vi "Set Variant.vi"(8 "error in (no error)":errorcluster, 10 "Variant":variant, 11 "int32 in":refnum<class "float.lvclass">) -> (0 "error out":errorcluster, 3 "int32 out":refnum<class "float.lvclass">)   [LabVIEW 2020, in "Protobuf RAW.lvlib" / "float.lvclass"]
uses:
  float.lvclass
  float.lvclass/float.ctl
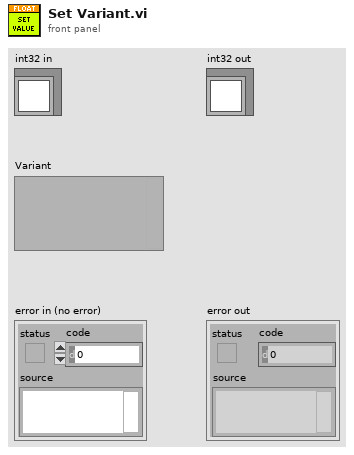
[diagram p1: front panel]
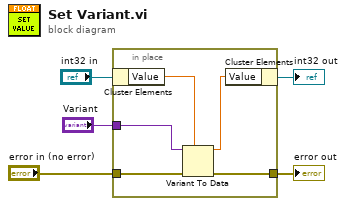
[diagram p0: block diagram]
diagram:
  n1 = in-place {
    in-place-border: "error in (no error)" -> [w10]
    in-place-border: [w9] -> w2
    in-place-border: "Variant" -> [w8]
    n2 = in-place-cluster #1("int32 in") -> ("Value"=w7:sgl)
    n3 = Variant To Data(error in=w10, type=w7, Variant=w8) -> (data=w6:sgl, error out=w9:errorcluster)
    n4 = in-place-cluster #1("Value"=w6) -> (→"int32 out":refnum<class "float.lvclass">)
  }
  "error out" <- w2
